vi "SendCommand.vi"(8 "error in (no error)":errorcluster, 10 "SubsystemData.lvclass":refnum<class "SubsystemData.lvclass">, 11 "Subsystem in":refnum<class "Subsystem.lvclass">) -> (0 "error out":errorcluster, 2 "queue out":refnum<queue>, 3 "Subsystem out":refnum<class "Subsystem.lvclass">)   [LabVIEW 2017, in "Subsystem.lvclass"]
uses:
  Subsystem.lvclass
  SubsystemData/SubsystemData.lvclass
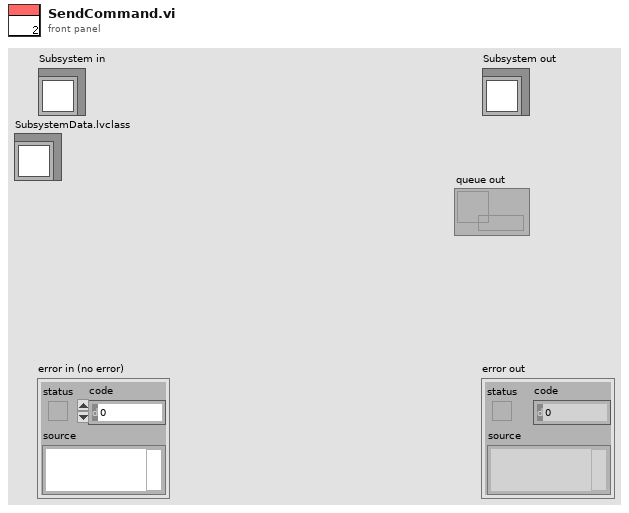
[diagram p1: front panel]
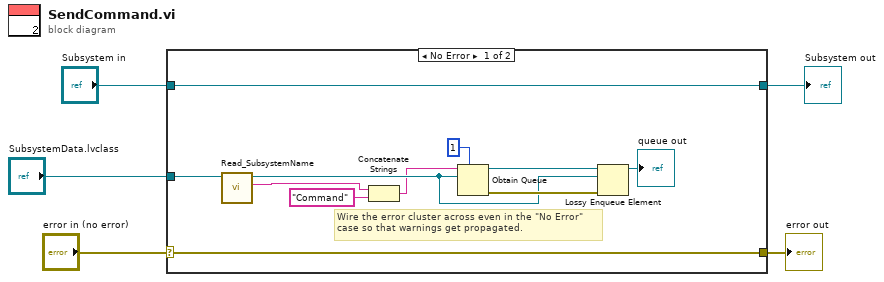
[diagram p0: block diagram]
diagram:
  n1 = case shown="No Error" "error in (no error)" {
    selector: "error in (no error)" -> [w16 w18]
    tunnel: [w16 w18] -> w4
    tunnel: [w12 w17] -> w2
    tunnel: "Subsystem in" -> [w12 w17]
    tunnel: "SubsystemData.lvclass" -> [w11 _]
    frame No Error {
      # "Wire the error cluster across even in the \"No Error\"\ncase so that warnings get propagated."
      n2 = call-dynamic "Read_SubsystemName.vi"("SubsystemData in"=w11) -> ("Subsystem Name"=w8:string, "SubsystemData out"=w10:refnum<class "SubsystemData.lvclass">)  [unwired: 8 in, 1 out]
      n3 = Concatenate Strings(w8, "Command") -> (w7:string)
      n4 = Obtain Queue(max queue size (-1, unlimited)=1, name (unnamed)=w7, element data type=w10) -> (queue out=w14:refnum<queue>, error out=w15:errorcluster)  [unwired: 2 in, 1 out]
      n5 = Lossy Enqueue Element(queue=w14, element=w10, error in (no error)=w15) -> (queue out=→"queue out":refnum<queue>)  [unwired: 3 out]
    }
    frame Error {
    }
  }
  "error out" <- w4
  "Subsystem out" <- w2
